vi "Print.vi"(0 "reference in":refnum<class "DataObject.lvclass">, 2 "String":string, 5 "error in (no error)":errorcluster) -> (14 "reference out":refnum<class "DataObject.lvclass">, 19 "error out":errorcluster)   [LabVIEW 2020, in "DataObject.lvclass"]
uses:
  DataObject.lvclass
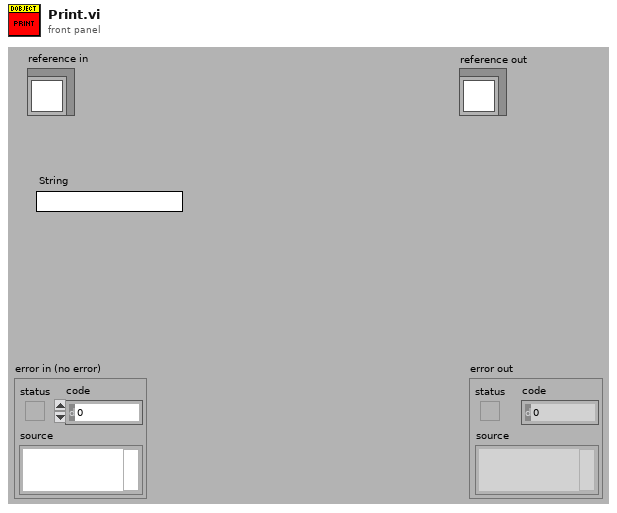
[diagram p1: front panel]
types:
  T1 = typedef "DataObject.lvclass/ObjectAttributes.ctl" = cluster{"StringRef":refnum<vi>}
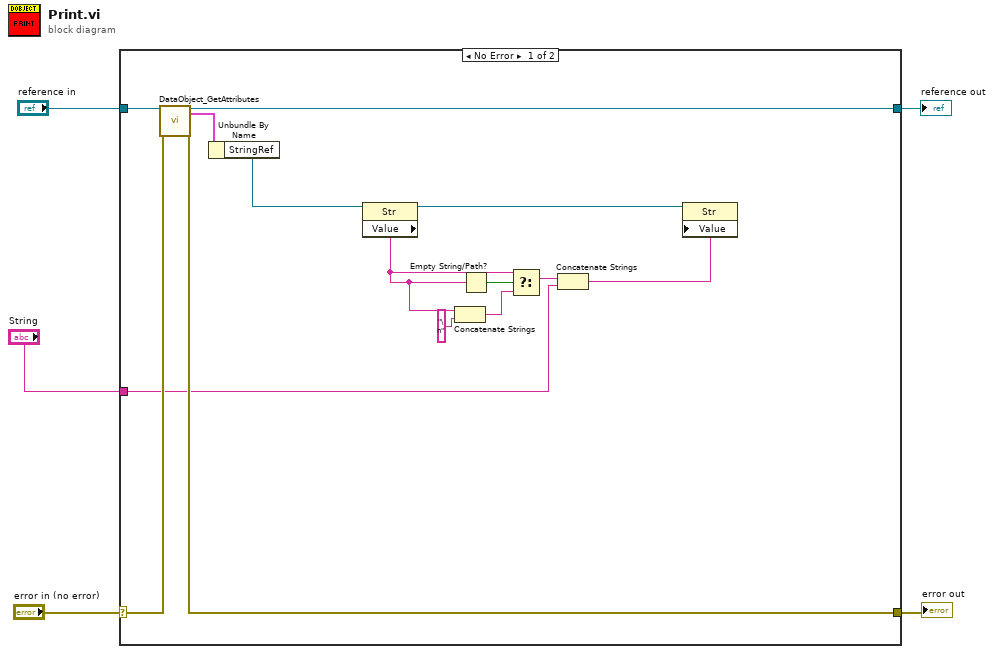
[diagram p0: block diagram]
diagram:
  n1 = case shown="No Error" "error in (no error)" {
    selector: "error in (no error)" -> [w19 w21]
    tunnel: [w17 w21] -> w4
    tunnel: [w15 w20] -> w2
    tunnel: "reference in" -> [w16 w20]
    tunnel: "String" -> [w7 _]
    frame No Error {
      n2 = call "DataObject_GetAttributes.vi"("reference in"=w16, "error in (no error)"=w19) -> ("reference out"=w15:refnum<class "DataObject.lvclass">, "Data"=w18:T1, "error out"=w17:errorcluster)  [unwired: 14 in, 1 out]
      n3 = Unbundle By Name(w18) -> ("StringRef"=w14:refnum<vi>)
      n4 = property class="Str"(reference=w14) -> (reference out=w13:refnum<vi>, "Value"=w11:string)  [unwired: 1 in, 1 out]
      n5 = Concatenate Strings(w11, "\n" ("string")) -> (w9:string)
      n6 = Empty String/Path?(string/path=w11) -> (empty?=w12:bool)
      n7 = Select(t=w11, s=w12, f=w9) -> (s? t:f=w8:string)
      n8 = Concatenate Strings(w8, w7) -> (w6:string)
      n9 = property class="Str"(reference=w13, "Value"=w6) -> ()  [unwired: 1 in, 2 out]
    }
    frame Error {
    }
  }
  "error out" <- w4
  "reference out" <- w2
